vi "copy project and open reference.vi"(8 "error in (no error)":errorcluster, 11 "project_folder":path) -> (0 "error out":errorcluster, 2 "root folder path":path, 3 "Project Ref out":refnum<vi>)   [LabVIEW 2024]
doc: "Copies the project to a random location on Temp folder and open the .lvproj that it finds under ./src folder"
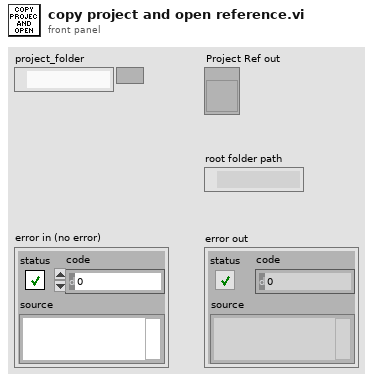
[diagram p1: front panel]
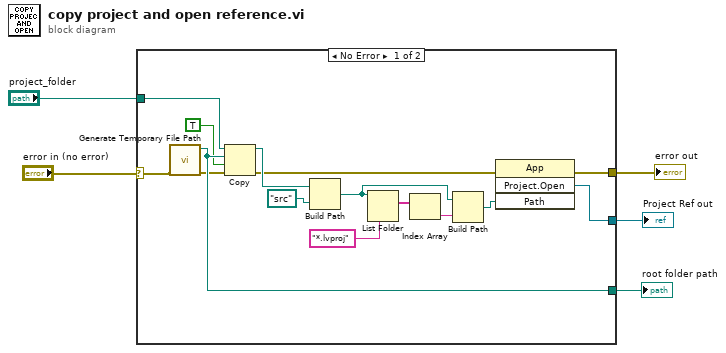
[diagram p0: block diagram]
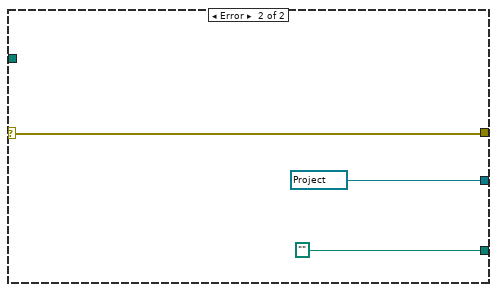
[diagram p2: hidden frame]
diagram:
  n1 = case shown="No Error" "error in (no error)" {
    selector: "error in (no error)" -> [w6 w23]
    tunnel: [w20 w23] -> w5
    tunnel: [w19 path "" ("Unique Temporary File Path")] -> w4
    tunnel: [w18 refnum<vi> refnum ("Project:Open")] -> w3
    tunnel: "project_folder" -> [w7 _]
    frame No Error {
      n2 = call <vilib>:"Generate Temporary File Path.vi"("error in (no error)"=w6) -> ("error out"=w14:errorcluster, "Unique Temporary File Path"=w19:path)  [unwired: 9 in]
      n3 = Copy(8:w14, 9:TRUE ("overwrite (F)"), 10:w19, 11:w7) -> (0:w15:errorcluster, 3:w17:path)  [unwired: 1 in, 1 out]
      n4 = Build Path(base path=w17, name or relative path=path "src") -> (appended path=w12:path)
      n5 = List Folder(path=w12, pattern="*.lvproj") -> (filenames=w10:string[])  [unwired: 2 in, 3 out]
      n6 = Index Array(array=w10) -> (element=w11:string)  [unwired: 1 in]
      n7 = Build Path(base path=w12, name or relative path=w11) -> (appended path=w13:path)
      n8 = invoke class="App" method="Project.Open"(error in=w15, "Path"=w13) -> (error out=w20:errorcluster, "Project:Open"=w18:refnum<vi>)  [unwired: 2 in, 2 out]
    }
    frame Error {
    }
  }
  "error out" <- w5
  "root folder path" <- w4
  "Project Ref out" <- w3
